vi "FlatToRichniswitch_grpc_RelayControlRequest.vi"(5 "OutputClusterType":T1, 11 "InputCluster":T3) -> (3 "OutputCluster":T1)   [LabVIEW 2021, in "NI Switch_client.lvlib"]
uses:
  NI Switch_client.lvlib
  niswitch_grpc_RelayControlRequest_relay_action_enum/niswitch_grpc_RelayControlRequest_relay_action_enum.lvclass
  nidevice_grpc_Session_session/nidevice_grpc_Session_session.lvclass
  nidevice_grpc_Session.ctl
  niswitch_grpc_RelayControlRequest.ctl
  niswitch_grpc_RelayAction.ctl
  nidevice_grpc_Session_Flat.ctl
  niswitch_grpc_RelayControlRequest_Flat.ctl
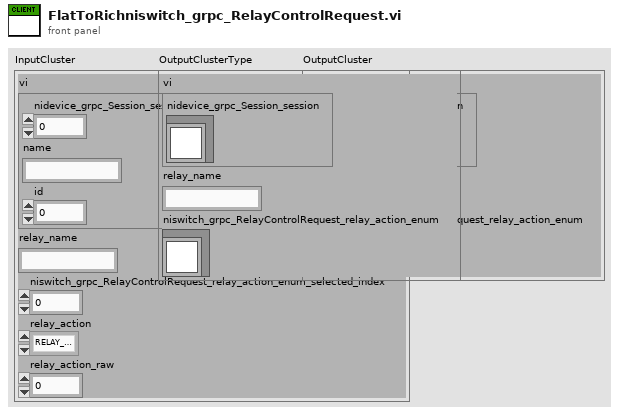
[diagram p1: front panel]
types:
  T1 = typedef "NI Switch_client.lvlib/niswitch_grpc_RelayControlRequest.ctl" = cluster{"vi":T2, "relay_name":string, "niswitch_grpc_RelayControlRequest_relay_action_enum":refnum<class "niswitch_grpc_RelayControlRequest_relay_action_enum.lvclass">}
  T2 = typedef "NI Switch_client.lvlib/nidevice_grpc_Session.ctl" = cluster{"nidevice_grpc_Session_session":refnum<class "nidevice_grpc_Session_session.lvclass">}
  T3 = typedef "NI Switch_client.lvlib/niswitch_grpc_RelayControlRequest_Flat.ctl" = cluster{"vi":T4, "relay_name":string, "niswitch_grpc_RelayControlRequest_relay_action_enum_selected_index":i32, "relay_action":T5, "relay_action_raw":i32}
  T4 = typedef "NI Switch_client.lvlib/nidevice_grpc_Session_Flat.ctl" = cluster{"nidevice_grpc_Session_session_selected_index":i32, "name":string, "id":u32}
  T5 = typedef "NI Switch_client.lvlib/niswitch_grpc_RelayAction.ctl" = enum32{"RELAY_ACTION_UNSPECIFIED", "RELAY_ACTION_NISWITCH_VAL_OPEN_RELAY", "RELAY_ACTION_NISWITCH_VAL_CLOSE_RELAY"}
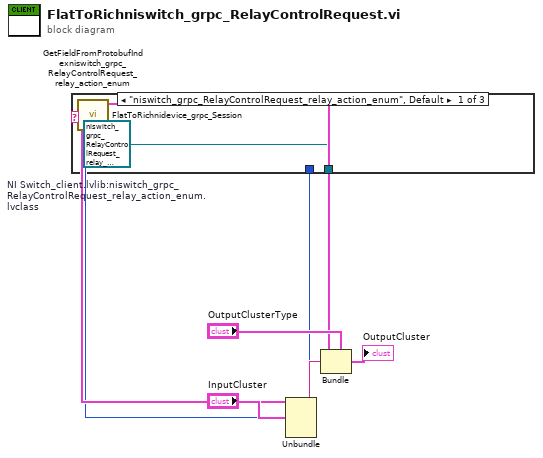
[diagram p0: block diagram]
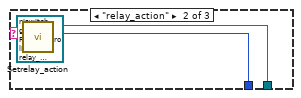
[diagram p2: hidden frame]
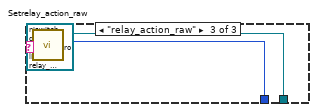
[diagram p3: hidden frame]
diagram:
  n1 = Unbundle "Unbundle"("InputCluster") -> ("vi"=w8:T4, "relay_name"=w6:string, "niswitch_grpc_RelayControlRequest_relay_action_enum_selected_index"=w5:i32, "relay_action"=w2:T5, "relay_action_raw"=w1:i32)
  n2 = call "GetFieldFromProtobufIndexniswitch_grpc_RelayControlRequest_relay_action_enum.vi"("protobuf index"=w5) -> ("oneof field name"=w4:string)
  n3 = case "niswitch_grpc_RelayControlRequest_relay_action_enum" shown="\"niswitch_grpc_RelayControlRequest_relay_action_enum\", Default" w4 {
    tunnel: [w12 w14 w17] -> w3
    tunnel: w2 -> [_ w15 _]
    tunnel: w1 -> [_ _ w18]
    frame "niswitch_grpc_RelayControlRequest_relay_action_enum", Default {
      w12 = refnum<class "niswitch_grpc_RelayControlRequest_relay_action_enum.lvclass"> refnum  # NI Switch_client.lvlib:niswitch_grpc_RelayControlRequest_relay_action_enum.lvclass
    }
    frame "relay_action" {
      n4 = call "Setrelay_action.vi"("Set_Val"=w15, "OneOfTemplate in"=refnum<class "niswitch_grpc_RelayControlRequest_relay_action_enum.lvclass"> refnum) -> ("OneOfTemplate out"=w14:refnum<class "niswitch_grpc_RelayControlRequest_relay_action_enum.lvclass">)  [unwired: 8 in, 1 out]
    }
    frame "relay_action_raw" {
      n5 = call "Setrelay_action_raw.vi"("Set_Val"=w18, "OneOfTemplate in"=refnum<class "niswitch_grpc_RelayControlRequest_relay_action_enum.lvclass"> refnum) -> ("OneOfTemplate out"=w17:refnum<class "niswitch_grpc_RelayControlRequest_relay_action_enum.lvclass">)  [unwired: 8 in, 1 out]
    }
  }
  n6 = call "FlatToRichnidevice_grpc_Session.vi"("InputCluster"=w8) -> ("OutputCluster"=w7:T2)  [unwired: 10 in]
  n7 = Bundle "Bundle"(cluster="OutputClusterType", "vi"=w7, "relay_name"=w6, "niswitch_grpc_RelayControlRequest_relay_action_enum"=w3) -> (→"OutputCluster":T1)
